vi "Configure Horizontal.vi"(8 "error in":errorcluster, 11 "Scope PXI CFG in":refnum<class "Scope PXI CFG.lvclass">) -> (0 "error out":errorcluster, 3 "Scope PXI CFG out":refnum<class "Scope PXI CFG.lvclass">)   [LabVIEW 2023, in "Scope.lvlib" / "Scope PXI.lvlib" / "Scope PXI CFG.lvclass"]
uses:
  Scope PXI CFG.lvclass
  Scope PXI CFG.lvclass/Scope PXI CFG.ctl
  Configuration Base/Configuration Base.lvclass/Configuration Base.ctl
  2f0dfe3b-727d-435f-a334-361c3472aed8.vi
  a8bb4bbf-f82b-4e58-9fc0-885d6d8595a7.vi
  2afd0b27-f59c-4e4c-ab34-d1b063ee1579.vi
  46d73ebe-6710-4003-86ab-c95650fc7a2a.vi
  88285a36-7fea-47d7-9b3a-47c90033b7a9.vi
  <vilib>/JDP Science/JSONtext/Next JSON Value.vi
  <vilib>/JDP Science/JSONtext/String Subset.vi
  <vilib>/JDP Science/JSONtext/Parsing/Advance past next JSON Value (inlined COPY).vi
  <vilib>/JDP Science/JSONtext/Parsing/Advance past whitespace.vi
  <vilib>/JDP Science/JSONtext/Parsing/Advance past String.vi
  <vilib>/JDP Science/JSONtext/Parsing/Advance past Number.vi
  <vilib>/JDP Science/JSONtext/Parsing/Advance past Line Ending.vi
  <vilib>/JDP Science/JSONtext/Parsing/Parse Full Path or Item Name.vi
  <vilib>/JDP Science/JSONtext/Parsing/Advance past Array.vi
  <vilib>/JDP Science/JSONtext/Parsing/Advance past Object.vi
  <vilib>/JDP Science/JSONtext/support/Error Cluster From Code.vi
  <vilib>/JDP Science/JSONtext/Offset/Find Item Locations by Path.vi
  <vilib>/JDP Science/JSONtext/JSON text to Variant.vi
  <vilib>/Utility/error.llb/Error Cluster From Error Code.vi
  <vilib>/JDP Science/JSONtext/LVClass Serializer/JSONtext LVClass Serializer.lvclass
  <vilib>/ErrorRing/Error Ring.xnode
  Configuration Base/Configuration Base.lvclass
  <vilib>/JDP Science/JSONtext/JSONtext.lvlib
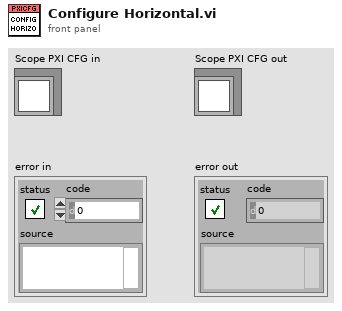
[diagram p1: front panel]
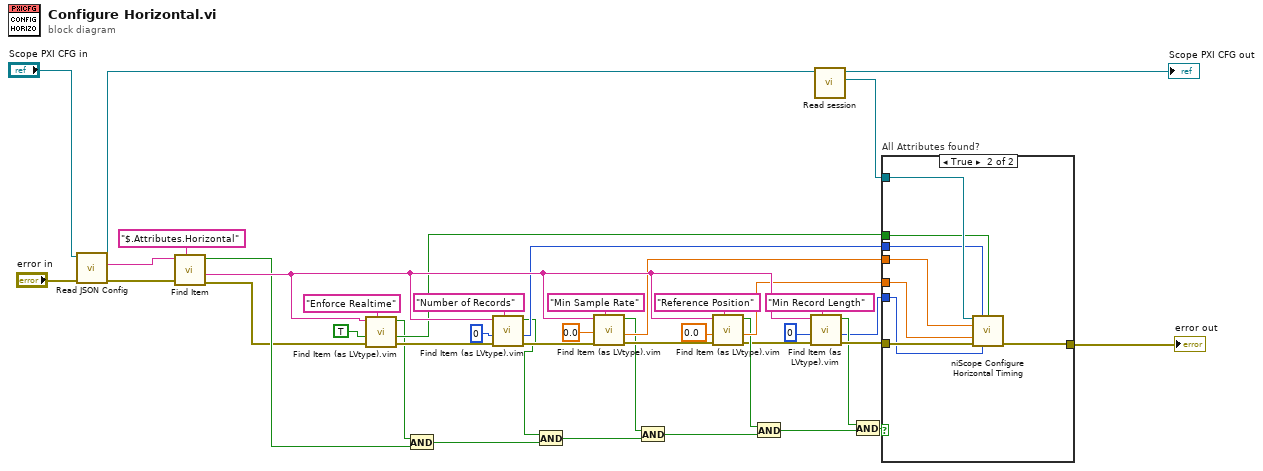
[diagram p0: block diagram]
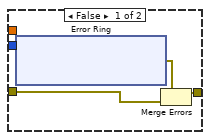
[diagram p2: hidden frame]
diagram:
  n1 = call "Read JSON Config.vi"("error in"="error in", "object in"="Scope PXI CFG in") -> ("error out"=w41:errorcluster, "<JSON>Config"=w33:string, "object out"=w34:refnum<class "Scope PXI CFG.lvclass">)  [unwired: 7 in]
  n2 = call <vilib>:"Find Item.vi"("$Path or Item Name"="$.Attributes.Horizontal", "error in (no error)"=w41, "JSON"=w33) -> ("error out"=w31:errorcluster, "<JSON>"=w40:string, "Found"=w32:bool)  [unwired: 5 in, 1 out]
  n3 = call "Find Item (as LVtype).vim"("$Path or Item Name"="Enforce Realtime", "error in (no error)"=w31, "Data Type and Default Value"=TRUE, "JSON"=w40) -> ("error out"=w27:errorcluster, "Data"=w26:bool, "Found"=w18:bool)  [unwired: 4 in, 1 out]
  n4 = And(x=w18, y=w32) -> (x .and. y?=w16:bool)
  n5 = call "Find Item (as LVtype).vim"("$Path or Item Name"="Number of Records", "error in (no error)"=w27, "Data Type and Default Value"=0, "JSON"=w40) -> ("error out"=w23:errorcluster, "Data"=w25:i32, "Found"=w17:bool)  [unwired: 4 in, 1 out]
  n6 = And(x=w17, y=w16) -> (x .and. y?=w14:bool)
  n7 = call "Find Item (as LVtype).vim"("$Path or Item Name"="Min Sample Rate", "error in (no error)"=w23, "Data Type and Default Value"=0.0, "JSON"=w40) -> ("error out"=w22:errorcluster, "Data"=w21:dbl, "Found"=w15:bool)  [unwired: 4 in, 1 out]
  n8 = And(x=w15, y=w14) -> (x .and. y?=w12:bool)
  n9 = call "Find Item (as LVtype).vim"("$Path or Item Name"="Reference Position", "error in (no error)"=w22, "Data Type and Default Value"=0.0, "JSON"=w40) -> ("error out"=w9:errorcluster, "Data"=w19:dbl, "Found"=w13:bool)  [unwired: 4 in, 1 out]
  n10 = And(x=w13, y=w12) -> (x .and. y?=w11:bool)
  n11 = call "Find Item (as LVtype).vim"("$Path or Item Name"="Min Record Length", "error in (no error)"=w9, "Data Type and Default Value"=0, "JSON"=w40) -> ("error out"=w7:errorcluster, "Data"=w5:i32, "Found"=w6:bool)  [unwired: 4 in, 1 out]
  n12 = call "Read session.vi"("Scope PXI CFG in"=w34) -> ("session"=w39:refnum<k15>, "Scope PXI CFG out"=→"Scope PXI CFG out":refnum<class "Scope PXI CFG.lvclass">)  [unwired: 8 in, 1 out]
  n13 = And(x=w6, y=w11) -> (x .and. y?=w8:bool)
  n14 = case "All Attributes found?" shown="True" w8 {
    tunnel: w7 -> [w43 w58]
    tunnel: w26 -> [_ w51]
    tunnel: w25 -> [_ w52]
    tunnel: [w44 w57] -> w36
    tunnel: w21 -> [_ w53]
    tunnel: w19 -> [_ w54]
    tunnel: w5 -> [_ w55]
    tunnel: w39 -> [_ w56]
    frame False {
      n15 = xnode "Error Ring"() -> ("error out"=w45:errorcluster)
      n16 = Merge Errors(w45, w43) -> (w44:errorcluster)
    }
    frame True {
      n17 = call <instrlib>:"niScope Configure Horizontal Timing.vi"("instrument handle"=w56, "number of records"=w52, "enforce realtime"=w51, "min sample rate"=w53, "reference position"=w54, "error in"=w58, "min record length"=w55) -> ("error out"=w57:errorcluster)  [unwired: 7 in, 1 out]
    }
  }
  "error out" <- w36
